vi "Add Caption and image.vi"(0 "PDF Report IN":refnum<class "PDF Report Class.lvclass">, 2 "Caption?":bool, 5 "Paragraph Refnum":refnum<k24>, 9 "Image Ref iTexSharp":refnum<k24>, 11 "error in (no error)":errorcluster) -> (4 "PDF Report OUT":refnum<class "PDF Report Class.lvclass">, 8 "Size (points)":cluster{"TotalHeight":sgl, "TotalWidth":sgl}, 15 "error out":errorcluster)   [LabVIEW 2019]
doc: "Version 1.0\nDeveloped by Jean-Marc Simard\nCopyright © 2010, Exaprom Inc.\nAll rights reserved.\nLicense: BSD\n\nWith iTextSharp 4.1.6 (http://itextsharp.sourceforge.net)\nunder Mozilla Public License Version 1.1\n(http://www.mozilla.org/MPL/MPL-1.1.html)"
uses:
  <userlib>/Exaprom PDF/LV Class/PDF Report Class/PDF Report Class.lvclass
  C:/Program Files/National Instruments/LabVIEW 2019/user.lib/Exaprom PDF/DLL/itextsharp.dll
  DLL/itextsharp.dll
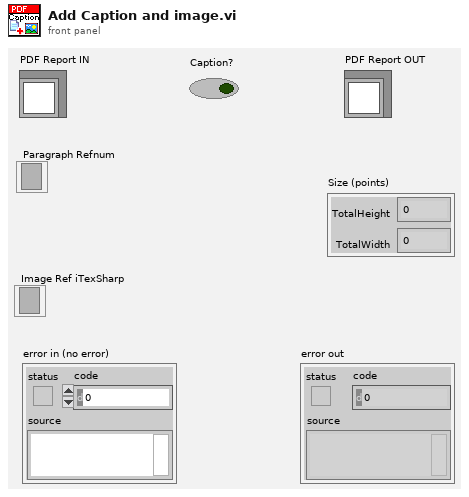
[diagram p1: front panel]
types:
  T1 = typedef "Captions.ctl" = cluster{"Figure":T2, "Table":T2, "Font":T3}
  T2 = typedef "Image or Table Caption.ctl" = cluster{"Caption":string, "Separator":string, "Position":enum16{"Above", "Below"}}
  T3 = typedef "Font complete cluster.ctl" = cluster{"Name":string, "Size":T4, "Color":T5, "Style":cluster{"Bold":bool, "Italic":bool, "Underline":bool, "Strikeout":bool}, "Type":T6}
  T4 = typedef "Font size.ctl" = sgl
  T5 = typedef "Font color.ctl" = u32
  T6 = typedef "Type and encoding.ctl" = cluster{"Type&direction":T7, "Embedded":bool, "Encoding":string}
  T7 = typedef "Type and run direction.ctl" = enum16{"Select", "ASCII", "UTF-16", "UTF-16 (default)", "UTF-16 (LTR)", "UTF-16 (RTL)"}
  T8 = cluster{"Captions":T1, "Image counter":u16, "Table counter":u16}
  T9 = typedef "Page dimensions.ctl" = cluster{"Start at page":i32, "Page Size":T10, "Orientation":T11, "widht":sgl, "height":sgl, "Margin left":sgl, "Margin right":sgl, "Margin top":sgl, "Margin bottom":sgl, "X0":sgl, "X1":sgl, "Y0":sgl, "Y1":sgl}
  T10 = typedef "Page size.ctl" = i32
  T11 = typedef "Page Orientation.ctl" = enum16{"Portrait", "Landscape"}
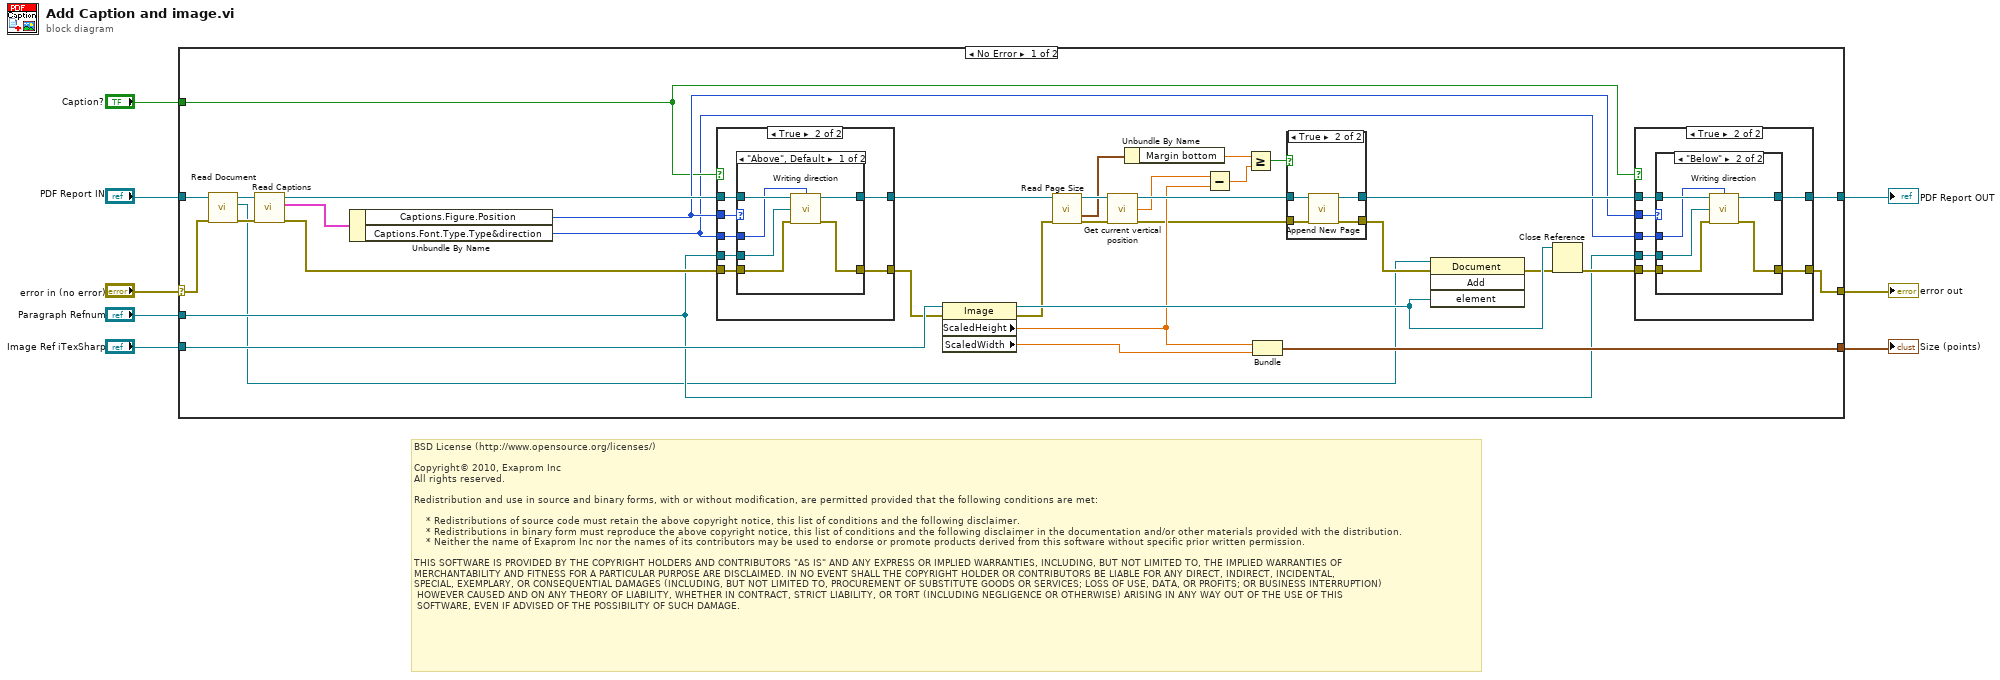
[diagram p0: block diagram]
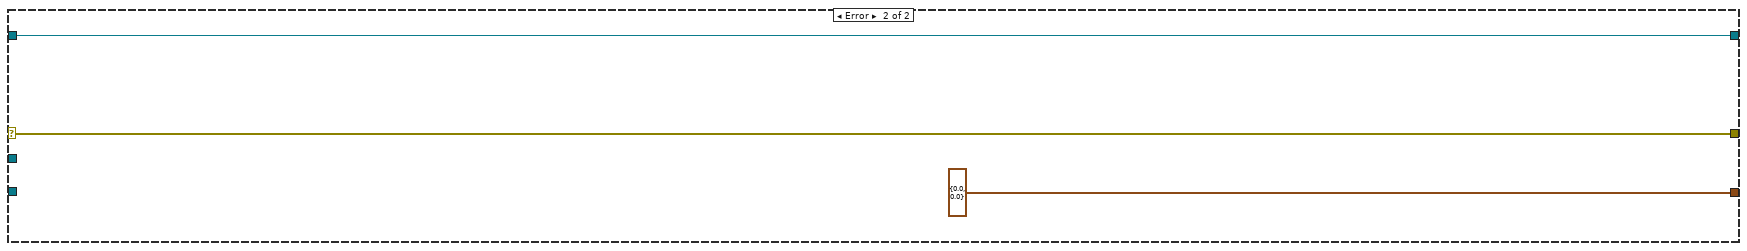
[diagram p7: hidden frame]
diagram:
  # "BSD License (http://www.opensource.org/licenses/)\n\nCopyright© 2010, Exaprom Inc\nAll rights reserved.\n\nRedistribution and use in source and binary forms, with or without modification, are permitted provided that the following conditions are met:\n\n    * Redistributions of source code must retain the above copyright notice, this list of conditions and the following disclaimer.\n    * Redistributions in binary form must reproduce the above copyright notice, this list of conditions and the following disclaimer in the documentation and/or other materials provided with the distribution.\n    * Neither the name of Exaprom Inc nor the names of its contributors may be used to endorse or promote products derived from this software without specific prior written permission.\n\nTHIS SOFTWARE IS PROVIDED BY THE COPYRIGHT HOLDERS AND CONTRIBUTORS \"AS IS\" AND ANY EXPRESS OR IMPLIED WARRANTIES, INCLUDING, BUT NOT LIMITED TO, THE IMPLIED WARRANTIES OF \nMERCHANTABILITY AND FITNESS FOR A PARTICULAR PURPOSE ARE DISCLAIMED. IN NO EVENT SHALL THE COPYRIGHT HOLDER OR CONTRIBUTORS BE LIABLE FOR ANY DIRECT, INDIRECT, INCIDENTAL,\nSPECIAL, EXEMPLARY, OR CONSEQUENTIAL DAMAGES (INCLUDING, BUT NOT LIMITED TO, PROCUREMENT OF SUBSTITUTE GOODS OR SERVICES; LOSS OF USE, DATA, OR PROFITS; OR BUSINESS INTERRUPTION)\n HOWEVER CAUSED AND ON ANY THEORY OF LIABILITY, WHETHER IN CONTRACT, STRICT LIABILITY, OR TORT (INCLUDING NEGLIGENCE OR OTHERWISE) ARISING IN ANY WAY OUT OF THE USE OF THIS\n SOFTWARE, EVEN IF ADVISED OF THE POSSIBILITY OF SUCH DAMAGE."
  n1 = case shown="No Error" "error in (no error)" {
    selector: "error in (no error)" -> [w21 w86]
    tunnel: "PDF Report IN" -> [w42 w85]
    tunnel: [w16 w85] -> w7
    tunnel: [w14 w86] -> w6
    tunnel: [w43 cluster{"ScaledHeight":sgl, "ScaledWidth":sgl} {"ScaledHeight"=0.0, "ScaledWidth"=0.0}] -> w3
    tunnel: "Image Ref iTexSharp" -> [w41 _]
    tunnel: "Caption?" -> [w12 _]
    tunnel: "Paragraph Refnum" -> [w11 _]
    frame No Error {
      n2 = call-dynamic "Read Document.vi"("error in (no error)"=w21, "PDF Report Class in"=w42) -> ("error out"=w22:errorcluster, "Document"=w10:refnum<k24>, "PDF Report Class out"=w24:refnum<class "PDF Report Class.lvclass">)  [unwired: 7 in]
      n3 = call-dynamic "Read Captions.vi"("error in (no error)"=w22, "PDF Report Class in"=w24) -> ("error out"=w20:errorcluster, "Captions and counters"=w23:T8, "PDF Report Class out"=w19:refnum<class "PDF Report Class.lvclass">)  [unwired: 7 in]
      n4 = Unbundle By Name(w23) -> ("Captions.Figure.Position"=w13:enum16{"Above", "Below"}, "Captions.Font.Type.Type&direction"=w9:T7)
      n5 = case shown="True" w12 {
        tunnel: w20 -> [w62 w69]
        tunnel: [w62 w68] -> w25
        tunnel: w13 -> [_ w67]
        tunnel: w11 -> [_ w66]
        tunnel: w19 -> [w61 w65]
        tunnel: [w61 w64] -> w18
        tunnel: w9 -> [_ w63]
        frame False {
        }
        frame True {
          n6 = case shown="\"Above\", Default" w67 {
            tunnel: w66 -> [w70 _]
            tunnel: w69 -> [w73 w77]
            tunnel: [w72 w77] -> w68
            tunnel: w65 -> [w75 w76]
            tunnel: [w74 w76] -> w64
            tunnel: w63 -> [w71 _]
            frame "Above", Default {
              n7 = call <userlib>:"Writing direction.vi"("PDF Report IN"=w75, "Text type"=w71, "Paragraph refnum"=w70, "error in (no error)"=w73) -> ("PDF Report OUT"=w74:refnum<class "PDF Report Class.lvclass">, "error out"=w72:errorcluster)  [unwired: 10 in]
            }
            frame "Below" {
            }
          }
        }
      }
      n8 = property class="Image"(reference=w41, error in=w25) -> (reference out=w40:refnum<k24>, error out=w31:errorcluster, "ScaledHeight"=w32:sgl, "ScaledWidth"=w39:sgl)
      n9 = call <userlib>:"Read Page Size.vi"("PDF Report"=w18, "error in (no error)"=w31) -> ("PDF Report duplicate"=w37:refnum<class "PDF Report Class.lvclass">, "Page (points)"=w35:T9, "error out"=w36:errorcluster)  [unwired: 11 out]
      n10 = call <userlib>:"Get current vertical position.vi"("PDF Report In"=w37, "error in (no error)"=w36) -> ("PDF Report duplicate"=w38:refnum<class "PDF Report Class.lvclass">, "GetVerticalPosition (points)"=w33:sgl, "error out"=w28:errorcluster)  [unwired: 1 in, 10 out]
      n11 = Unbundle By Name(w35) -> ("Margin bottom"=w34:sgl)
      n12 = Subtract(x=w33, y=w32) -> (x-y=w30:sgl)
      n13 = Greater Or Equal?(x=w34, y=w30) -> (x >= y?=w29:bool)
      n14 = Bundle("ScaledHeight"=w32, "ScaledWidth"=w39) -> (w43:cluster{"ScaledHeight":sgl, "ScaledWidth":sgl})  [unwired: 1 out]
      n15 = case shown="True" w29 {
        tunnel: w38 -> [w79 w83]
        tunnel: [w79 w82] -> w17
        tunnel: w28 -> [w78 w81]
        tunnel: [w78 w80] -> w27
        frame False {
        }
        frame True {
          n16 = call <userlib>:"Append New Page.vi"("PDF Report"=w83, "error in (no error)"=w81) -> ("PDF Report duplicate"=w82:refnum<class "PDF Report Class.lvclass">, "error OUT"=w80:errorcluster)  [unwired: 12 out]
        }
      }
      n17 = invoke class="Document" method="Add"(reference=w10, error in=w27, "element"=w40) -> (error out=w26:errorcluster)  [unwired: 1 in, 3 out]
      n18 = Close Reference(reference=w40, error in (no error)=w26) -> (error out=w15:errorcluster)
      n19 = case shown="True" w12 {
        tunnel: w15 -> [w45 w52]
        tunnel: [w45 w51] -> w14
        tunnel: w13 -> [_ w50]
        tunnel: w11 -> [_ w49]
        tunnel: w17 -> [w44 w48]
        tunnel: [w44 w47] -> w16
        tunnel: w9 -> [_ w46]
        frame False {
        }
        frame True {
          n20 = case shown="\"Below\"" w50 {
            tunnel: w49 -> [_ w55]
            tunnel: w52 -> [w54 w58]
            tunnel: [w54 w57] -> w51
            tunnel: w48 -> [w53 w60]
            tunnel: [w53 w59] -> w47
            tunnel: w46 -> [_ w56]
            frame "Above", Default {
            }
            frame "Below" {
              n21 = call <userlib>:"Writing direction.vi"("PDF Report IN"=w60, "Text type"=w56, "Paragraph refnum"=w55, "error in (no error)"=w58) -> ("PDF Report OUT"=w59:refnum<class "PDF Report Class.lvclass">, "error out"=w57:errorcluster)  [unwired: 10 in]
            }
          }
        }
      }
    }
    frame Error {
    }
  }
  "PDF Report OUT" <- w7
  "error out" <- w6
  "Size (points)" <- w3
